vi "AcquireTransducerRingTime.vi"(9 "Cut-Off Level":dbl=1.0 format="%.2g", 11 "Ring Time Wavefrom Array":waveform(dbl)[](array[waveform])) -> (1 "RT Index":i32, 2 "Ring Time (ms)":dbl format="%.5g", 3 "Ring Time Wavefrom":waveform(dbl)(graph) caption="Ring Time Plot")   [LabVIEW 2019, in "Acquisition.lvlib"]
uses:
  Acquisition.lvlib
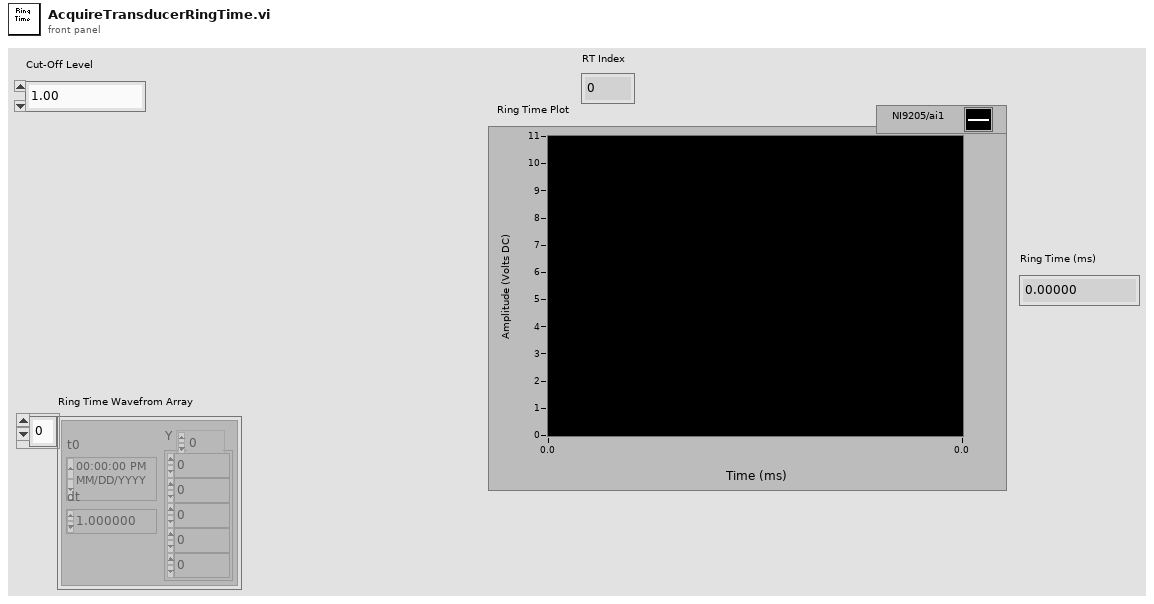
[diagram p1: front panel]
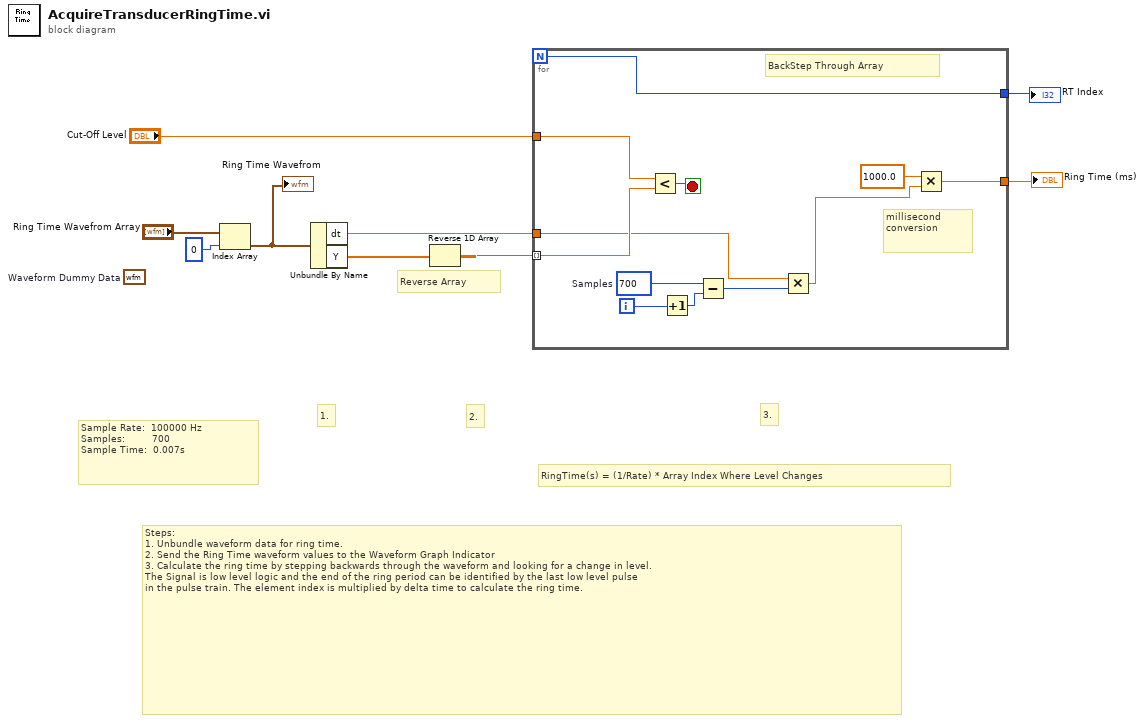
[diagram p0: block diagram]
diagram:
  (unwired) waveform(dbl) {"t0"=timestamp(3673525335.890183 s since 1904-01-01), "dt"=9.999999999999972e-06, "Y"=array[700 elements], "attributes"=variant("NI_ChannelName"=variant(string "NI9205/ai1"), "NI_UnitDescription"=variant(string "Volts"))}  # Waveform Dummy Data
  # "Reverse Array"
  # "Sample Rate:  100000 Hz\nSamples:         700\nSample Time:  0.007s"
  # "RingTime(s) = (1/Rate) * Array Index Where Level Changes"
  # "Steps: \n1. Unbundle waveform data for ring time.\n2. Send the Ring Time waveform values to the Waveform Graph Indicator\n3. Calculate the ring time by stepping backwards through the waveform and looking for a change in level.\nThe Signal is low level logic and the end of the ring period can be identified by the last low level pulse\nin the pulse train. The element index is multiplied by delta time to calculate the ring time."
  # "3."
  # "2."
  # "1."
  n1 = Index Array(array="Ring Time Wavefrom Array", index=0) -> (element=w5:waveform(dbl))
  "Ring Time Wavefrom" <- w5
  n2 = Unbundle By Name(w5) -> ("dt"=w1:dbl, "Y"=w4:dbl[])
  n3 = Reverse 1D Array(array=w4) -> (reversed array=w3:dbl[])
  n4 = for {
    N -> [w21]
    tunnel: "Cut-Off Level" -> [w20]
    tunnel: [w21] -> w7
    tunnel: w3 -> [w19] mode=indexing
    tunnel: [w10] -> w2
    tunnel: w1 -> [w13]
    i -> [w16]
    stop <- w18 stop-if-true
    w17 = 700  # Samples
    # "millisecond \nconversion"
    # "BackStep Through Array"
    n5 = Less?(x=w20, y=w19) -> (x < y?=w18:bool)
    n6 = Increment(x=w16) -> (x+1=w15:i32)
    n7 = Subtract(x=w17, y=w15) -> (x-y=w14:i32)
    n8 = Multiply(x=w13, y=w14) -> (x*y=w12:dbl)
    n9 = Multiply(x=1000.0, y=w12) -> (x*y=w10:dbl)
  }
  "RT Index" <- w7
  "Ring Time (ms)" <- w2
